vi "CRYPEAQ enThresh.vi"(11 "f":dbl[](array[numeric])) -> (3 "Et(thres)":dbl[](array[numeric]))   [LabVIEW 2013]
panel:
  out "XY Graph 2":cluster{"Center Frequency":dbl[], dbl[]}(graph)
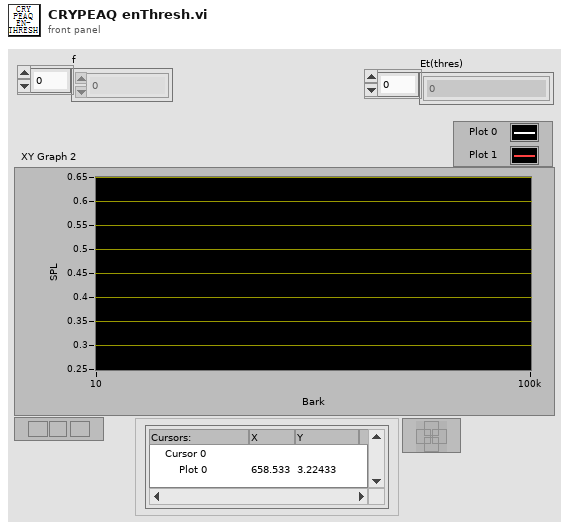
[diagram p1: front panel]
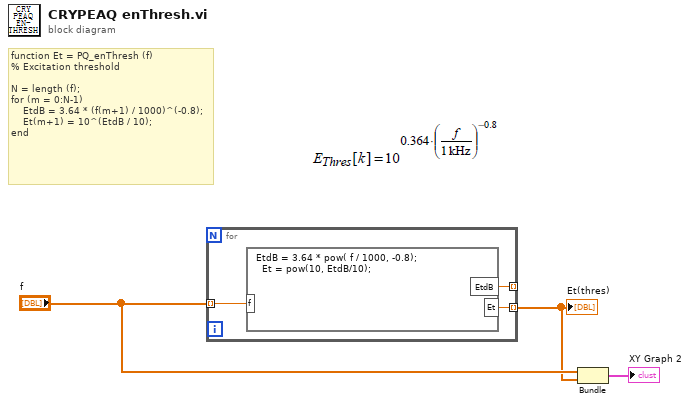
[diagram p0: block diagram]
diagram:
  # "function Et = PQ_enThresh (f)\n% Excitation threshold\n\nN = length (f);\nfor (m = 0:N-1)\n    EtdB = 3.64 * (f(m+1) / 1000)^(-0.8);\n    Et(m+1) = 10^(EtdB / 10);\nend"
  n1 = for {
    tunnel: "f" -> [w6] mode=indexing
    tunnel: [w5] -> _ mode=indexing
    tunnel: [w4] -> w1 mode=indexing
    n2 = formula code="EtdB = 3.64 * pow( f / 1000, -0.8);\n  Et = pow(10, EtdB/10);"("f"=w6) -> ("EtdB"=w5:dbl, "Et"=w4:dbl)
  }
  "Et(thres)" <- w1
  n3 = Bundle("f"="f", w1) -> (→"XY Graph 2":cluster{"f":dbl[], dbl[]})  [unwired: 1 in]
